vi "Nfocus driver V0.2.vi"(5 "error in":errorcluster, 8 "Refs In":T1) -> (0 "error out":errorcluster)   [LabVIEW 2016]
panel:
  out "Running":bool
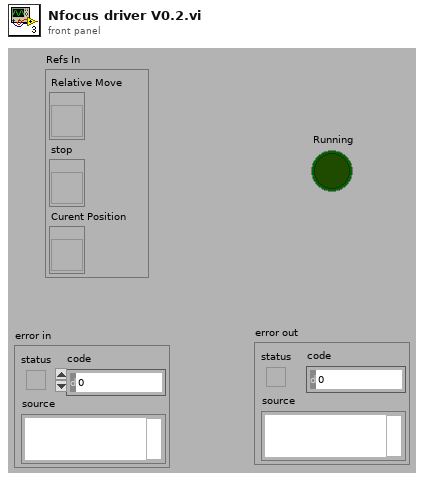
[diagram p1: front panel]
types:
  T1 = cluster{"Relative Move":refnum<vi>, "stop":refnum<vi>, "Curent Position ":refnum<vi>}
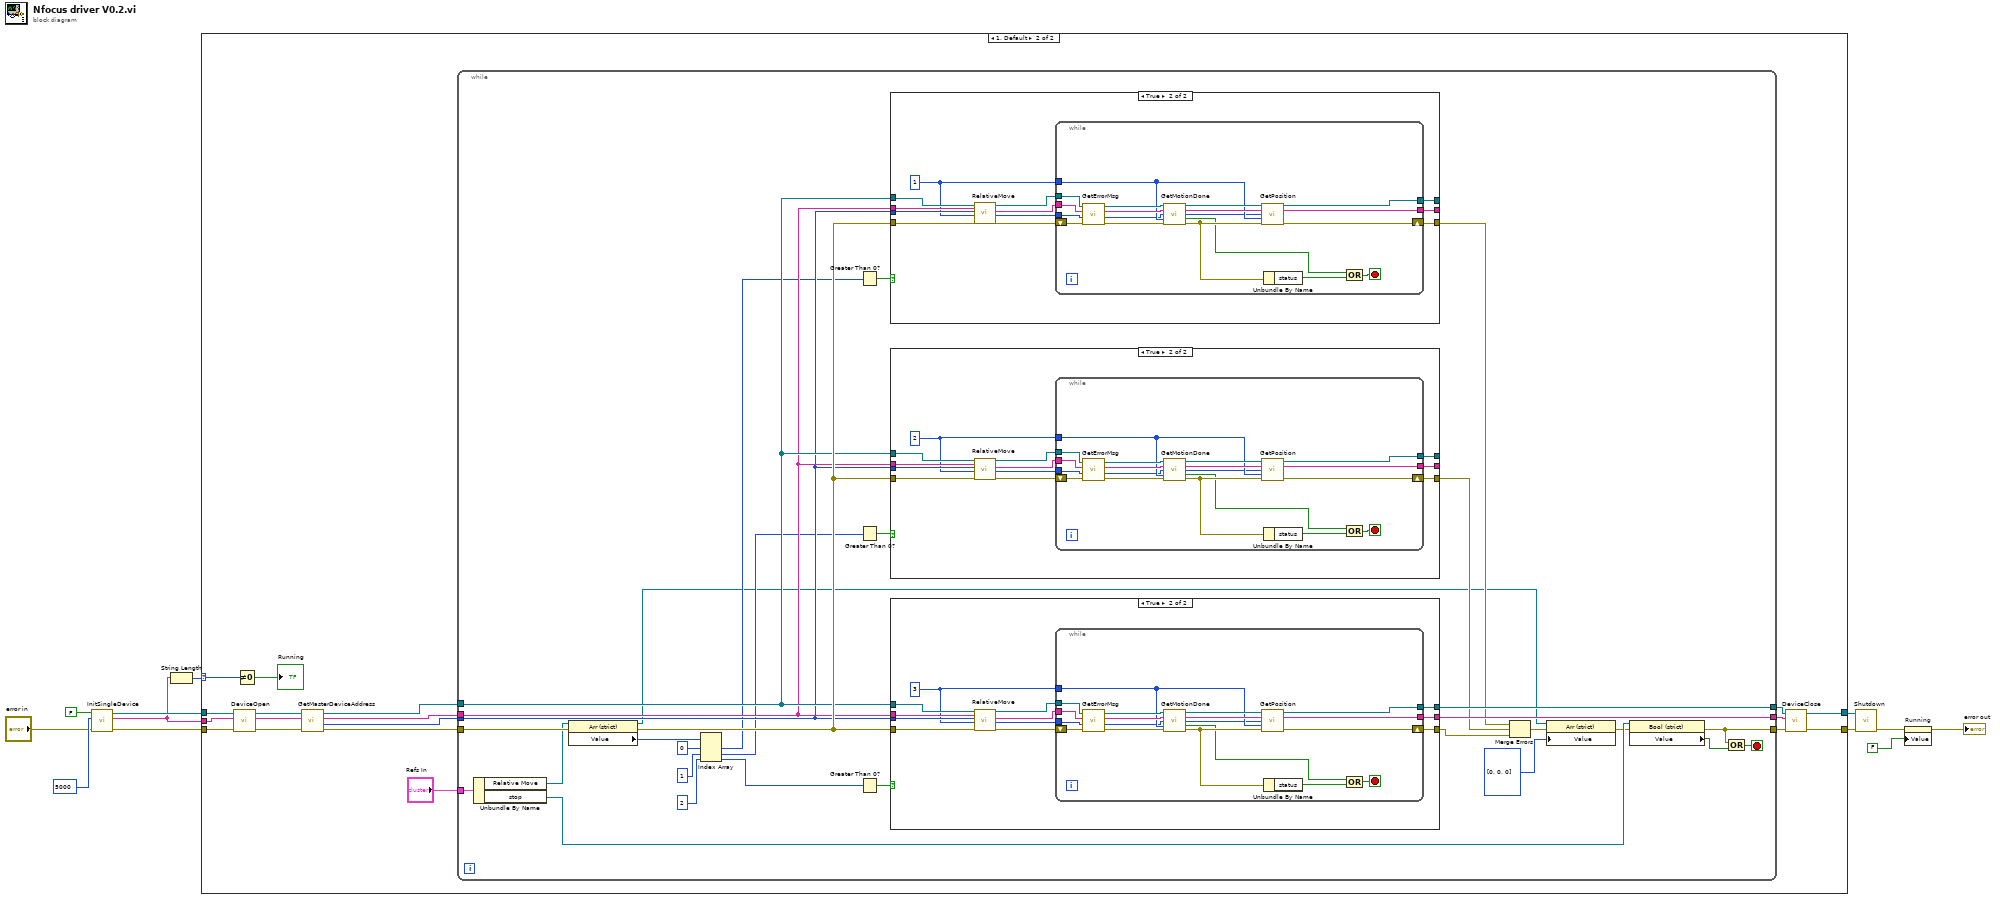
[diagram p0: block diagram]
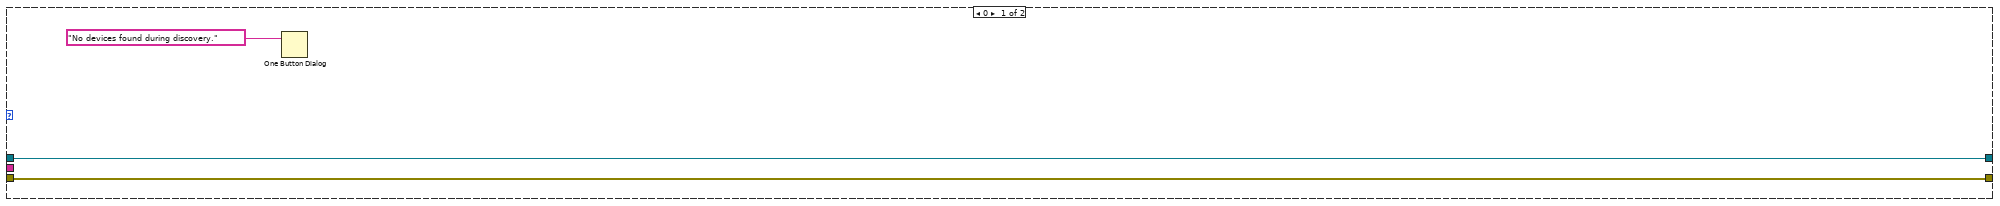
[diagram p2: hidden frame]
diagram:
  n1 = call "InitSingleDevice.vi"("error in (no error)"="error in", "msecDelayForDiscovery"=5000, "logging"=FALSE) -> ("error out"=w5:errorcluster, "DeviceKey Out"=w6:string, "CmdLib Out"=w8:refnum<k24>)  [unwired: 2 in]
  n2 = String Length(string=w6) -> (length=w7:i32)
  n3 = case shown="1, Default" w7 {
    selector: w7 -> [_ w18]
    tunnel: [w14 w20] -> w10
    tunnel: [w13 w22] -> w9
    tunnel: w8 -> [w14 w26]
    tunnel: w6 -> [_ w28]
    tunnel: w5 -> [w13 w30]
    frame 0 {
      n4 = One Button Dialog(message="No devices found during discovery.") -> ()  [unwired: 1 in, 1 out]
    }
    frame 1, Default {
      n5 = call "DeviceOpen.vi"("error in (no error)"=w30, "DeviceKey In"=w28, "CmdLib In"=w26) -> ("error out"=w29:errorcluster, "DeviceKey Out"=w27:string, "CmdLib Out"=w25:refnum<k24>)  [unwired: 2 in]
      n6 = Not Equal To 0?(x=w18) -> (x != 0?=→"Running":bool)
      n7 = call "GetMasterDeviceAddress.vi"("error in (no error)"=w29, "DeviceKey In"=w27, "CmdLib In"=w25) -> ("error out"=w19:errorcluster, "Device Address"=w33:i32, "DeviceKey Out"=w31:string, "CmdLib Out"=w32:refnum<k24>)  [unwired: 1 in]
      n8 = while {
        tunnel: w33 -> [w51]
        tunnel: w32 -> [w53]
        tunnel: [w62] -> w21
        tunnel: w19 -> [w55]
        tunnel: [w60] -> w23
        tunnel: w31 -> [w52]
        tunnel: [w63] -> w24
        tunnel: "Refs In" -> [w38]
        stop <- w61 stop-if-true
        n9 = Unbundle By Name(w38) -> ("Relative Move"=w40:refnum<vi>, "stop"=w39:refnum<vi>)
        n10 = property class="Arr (strict)"(reference=w40, error in=w55) -> (reference out=w35:refnum<vi>, error out=w54:errorcluster, "Value"=w57:i32[])
        n11 = Index Array(array=w57, index #1=0 ("index"), index #2=1 ("index"), index #3=2 ("index")) -> (element #1=w46:i32, element #2=w45:i32, element #3=w44:i32)
        n12 = Greater Than 0?(x=w46) -> (x > 0?=w47:bool)
        n13 = Greater Than 0?(x=w45) -> (x > 0?=w48:bool)
        n14 = Greater Than 0?(x=w44) -> (x > 0?=w58:bool)
        n15 = case shown="True" w47 {
          tunnel: w51 -> [_ w78]
          tunnel: w53 -> [w66 w77]
          tunnel: w52 -> [w65 w76]
          tunnel: [w65 w75] -> _
          tunnel: [w66 w74] -> _
          tunnel: w54 -> [w64 w73]
          tunnel: [w64 w72] -> w43
          frame False {
          }
          frame True {
            w67 = 1
            n16 = call "RelativeMove.vi"("CmdLib In"=w77, "DeviceKey In"=w76, "Device Address In"=w78, "Motor"=w67, "error in (no error)"=w73) -> ("CmdLib Out"=w71:refnum<k24>, "DeviceKey Out"=w70:string, "Device Address Out"=w68:i32, "error out"=w69:errorcluster)  [unwired: 11 in]
            n17 = while {
              tunnel: w67 -> [w93]
              tunnel: w71 -> [w92]
              tunnel: w70 -> [w91]
              tunnel: [w86] -> w74
              tunnel: w68 -> [w85]
              shift-right: [w87] -> w72
              shift-left: w69 -> [w90]
              tunnel: [w82] -> w75
              stop <- w81 stop-if-true
              n18 = call "GetErrorMsg.vi"("error in (no error)"=w90, "Device Address In"=w85, "DeviceKey In"=w91, "CmdLib In"=w92) -> ("error out"=w89:errorcluster, "Device Address Out"=w84:i32, "DeviceKey Out"=w95:string, "CmdLib Out"=w94:refnum<k24>)
              n19 = call "GetMotionDone.vi"("CmdLib In"=w94, "DeviceKey In"=w95, "Device Address In"=w84, "Motor"=w93, "error in (no error)"=w89) -> ("CmdLib Out"=w96:refnum<k24>, "DeviceKey Out"=w97:string, "Device Address Out"=w83:i32, "Is Motion Done"=w80:bool, "error out"=w88:errorcluster)  [unwired: 6 in]
              n20 = call "GetPosition.vi"("CmdLib In"=w96, "DeviceKey In"=w97, "Device Address In"=w83, "Motor"=w93, "error in (no error)"=w88) -> ("CmdLib Out"=w86:refnum<k24>, "DeviceKey Out"=w82:string, "error out"=w87:errorcluster)  [unwired: 6 in, 2 out]
              n21 = Unbundle By Name(w88) -> ("status"=w79:bool)
              n22 = Compound Arithmetic op=OR(w80, w79) -> (w81:bool)
            }
          }
        }
        n23 = case shown="True" w48 {
          tunnel: w51 -> [_ w112]
          tunnel: w53 -> [w100 w111]
          tunnel: w52 -> [w99 w110]
          tunnel: [w99 w109] -> _
          tunnel: [w100 w108] -> _
          tunnel: w54 -> [w98 w107]
          tunnel: [w98 w106] -> w42
          frame False {
          }
          frame True {
            w101 = 2
            n24 = call "RelativeMove.vi"("CmdLib In"=w111, "DeviceKey In"=w110, "Device Address In"=w112, "Motor"=w101, "error in (no error)"=w107) -> ("CmdLib Out"=w105:refnum<k24>, "DeviceKey Out"=w104:string, "Device Address Out"=w102:i32, "error out"=w103:errorcluster)  [unwired: 11 in]
            n25 = while {
              tunnel: w101 -> [w127]
              tunnel: w105 -> [w126]
              tunnel: w104 -> [w125]
              tunnel: [w120] -> w108
              tunnel: w102 -> [w119]
              shift-right: [w121] -> w106
              shift-left: w103 -> [w124]
              tunnel: [w116] -> w109
              stop <- w115 stop-if-true
              n26 = call "GetErrorMsg.vi"("error in (no error)"=w124, "Device Address In"=w119, "DeviceKey In"=w125, "CmdLib In"=w126) -> ("error out"=w123:errorcluster, "Device Address Out"=w118:i32, "DeviceKey Out"=w129:string, "CmdLib Out"=w128:refnum<k24>)
              n27 = call "GetMotionDone.vi"("CmdLib In"=w128, "DeviceKey In"=w129, "Device Address In"=w118, "Motor"=w127, "error in (no error)"=w123) -> ("CmdLib Out"=w130:refnum<k24>, "DeviceKey Out"=w131:string, "Device Address Out"=w117:i32, "Is Motion Done"=w114:bool, "error out"=w122:errorcluster)  [unwired: 6 in]
              n28 = call "GetPosition.vi"("CmdLib In"=w130, "DeviceKey In"=w131, "Device Address In"=w117, "Motor"=w127, "error in (no error)"=w122) -> ("CmdLib Out"=w120:refnum<k24>, "DeviceKey Out"=w116:string, "error out"=w121:errorcluster)  [unwired: 6 in, 2 out]
              n29 = Unbundle By Name(w122) -> ("status"=w113:bool)
              n30 = Compound Arithmetic op=OR(w114, w113) -> (w115:bool)
            }
          }
        }
        n31 = case shown="True" w58 {
          tunnel: w51 -> [_ w146]
          tunnel: w53 -> [w134 w145]
          tunnel: w52 -> [w133 w144]
          tunnel: [w133 w143] -> w63
          tunnel: [w134 w142] -> w62
          tunnel: w54 -> [w132 w141]
          tunnel: [w132 w140] -> w41
          frame False {
          }
          frame True {
            w135 = 3
            n32 = call "RelativeMove.vi"("CmdLib In"=w145, "DeviceKey In"=w144, "Device Address In"=w146, "Motor"=w135, "error in (no error)"=w141) -> ("CmdLib Out"=w139:refnum<k24>, "DeviceKey Out"=w138:string, "Device Address Out"=w136:i32, "error out"=w137:errorcluster)  [unwired: 11 in]
            n33 = while {
              tunnel: w135 -> [w161]
              tunnel: w139 -> [w160]
              tunnel: w138 -> [w159]
              tunnel: [w154] -> w142
              tunnel: w136 -> [w153]
              shift-right: [w155] -> w140
              shift-left: w137 -> [w158]
              tunnel: [w150] -> w143
              stop <- w149 stop-if-true
              n34 = call "GetErrorMsg.vi"("error in (no error)"=w158, "Device Address In"=w153, "DeviceKey In"=w159, "CmdLib In"=w160) -> ("error out"=w157:errorcluster, "Device Address Out"=w152:i32, "DeviceKey Out"=w163:string, "CmdLib Out"=w162:refnum<k24>)
              n35 = call "GetMotionDone.vi"("CmdLib In"=w162, "DeviceKey In"=w163, "Device Address In"=w152, "Motor"=w161, "error in (no error)"=w157) -> ("CmdLib Out"=w164:refnum<k24>, "DeviceKey Out"=w165:string, "Device Address Out"=w151:i32, "Is Motion Done"=w148:bool, "error out"=w156:errorcluster)  [unwired: 6 in]
              n36 = call "GetPosition.vi"("CmdLib In"=w164, "DeviceKey In"=w165, "Device Address In"=w151, "Motor"=w161, "error in (no error)"=w156) -> ("CmdLib Out"=w154:refnum<k24>, "DeviceKey Out"=w150:string, "error out"=w155:errorcluster)  [unwired: 6 in, 2 out]
              n37 = Unbundle By Name(w156) -> ("status"=w147:bool)
              n38 = Compound Arithmetic op=OR(w148, w147) -> (w149:bool)
            }
          }
        }
        n39 = Merge Errors(w43, w42, w41) -> (w36:errorcluster)
        n40 = property class="Arr (strict)"(reference=w35, error in=w36, "Value"=i32[] [0, 0, 0]) -> (error out=w37:errorcluster)  [unwired: 1 out]
        n41 = property on="Property Node" class="Bool (strict)"(reference=w39, error in=w37) -> (error out=w60:errorcluster, "Value"=w59:bool)  [unwired: 1 out]
        n42 = Compound Arithmetic op=OR(w60, w59) -> (w61:bool)
      }
      n43 = call "DeviceClose.vi"("error in (no error)"=w23, "DeviceKey In"=w24, "CmdLib In"=w21) -> ("error out"=w22:errorcluster, "CmdLib Out"=w20:refnum<k24>)  [unwired: 2 in, 1 out]
    }
  }
  n44 = call "Shutdown.vi"("error in (no error)"=w9, "CmdLib In"=w10) -> ("error out"=w3:errorcluster)  [unwired: 4 in, 1 out]
  n45 = property on="Running" class="Bool (strict)"(error in=w3, "Value"=FALSE ("Boolean")) -> (error out=→"error out":errorcluster)  [unwired: 1 in, 1 out]
